vi "UpdateProject.vi"(8 "error in (no error)":errorcluster, 11 "DB_SQLite in":refnum<class "DB_SQLite.lvclass">) -> (0 "error out":errorcluster, 3 "DB_SQLite out":refnum<class "DB_SQLite.lvclass">)   [LabVIEW 2020, in "DB_SQLite.lvclass"]
uses:
  DB_SQLite.lvclass
  C:/dev/TRANCON/Classes/DB/DB.lvclass
  DB.lvclass/DB.ctl
  <vilib>/drjdpowell/SQLite Library/SQL Statement/SQL Statement.lvclass/SQL Statement.ctl
  <vilib>/drjdpowell/SQLite Library/SQL Statement/Bind Text.vi
  <vilib>/drjdpowell/SQLite Library/SQL Statement/Step.vi
  <vilib>/drjdpowell/SQLite Library/SQL Statement/Error Message.vi
  <vilib>/drjdpowell/SQLite Library/SQL Connection/Connection.lvclass
  <vilib>/drjdpowell/SQLite Library/SQL Statement/SQL Statement.lvclass
  <vilib>/drjdpowell/SQLite Library/Transaction Helpers/Transaction.lvlib
  DB.lvclass
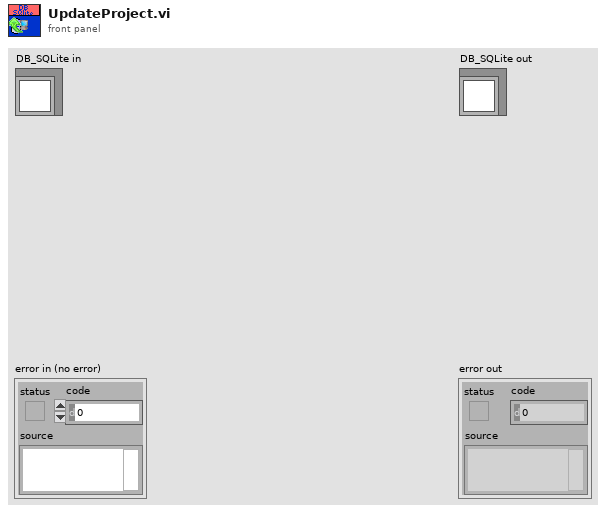
[diagram p1: front panel]
types:
  T1 = typedef "DB.lvclass/Def_DB_FP_ref_commands.ctl" = cluster{"Project Name":refnum<vi>, "Projects":refnum<vi>, "Project Description":refnum<vi>, "Project Date":refnum<vi>, "Project Users":refnum<vi>, "Samples":refnum<vi>, "Sample Name":refnum<vi>, "Sample Description":refnum<vi>, "Sample Date":refnum<vi>, "Experiments":refnum<vi>, "Exp Name":refnum<vi>, "Exp Description":refnum<vi>, "Exp Date":refnum<vi>, "Users":refnum<vi>, "User Name":refnum<vi>, "User Description":refnum<vi>, "User Date":refnum<vi>}
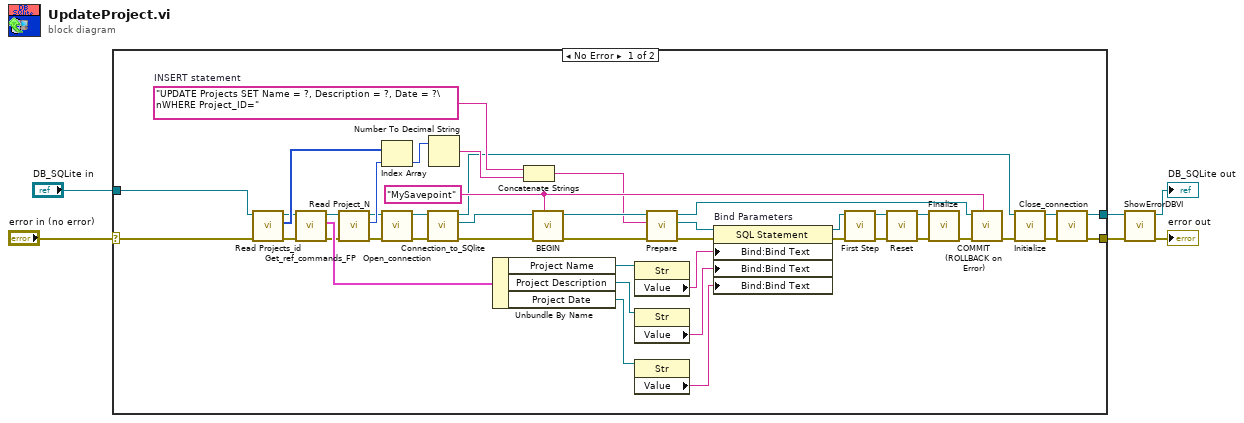
[diagram p0: block diagram]
diagram:
  n1 = case shown="No Error" "error in (no error)" {
    selector: "error in (no error)" -> [w19 w52]
    tunnel: [w12 w52] -> w3
    tunnel: [w11 w51] -> w4
    tunnel: "DB_SQLite in" -> [w23 w51]
    frame No Error {
      w44 = "MySavepoint" ("Savepoint name")
      w36 = "UPDATE Projects SET Name = ?, Description = ?, Date = ?\nWHERE Project_ID="  # INSERT statement
      n2 = call "Read Projects_id.vi"("error in (no error)"=w19, "DB in"=w23) -> ("error out"=w20:errorcluster, "Projects_id"=w22:i32[], "DB out"=w21:refnum<class "DB_SQLite.lvclass">)  [unwired: 7 in]
      n3 = call "Get_ref_commands_FP.vi"("error in (no error)"=w20, "DB in"=w21) -> ("error out"=w24:errorcluster, "controls_refs"=w25:T1, "DB out"=w26:refnum<class "DB_SQLite.lvclass">)  [unwired: 7 in]
      n4 = call "Read Project_N.vi"("error in (no error)"=w24, "DB in"=w26) -> ("error out"=w15:errorcluster, "Project_N"=w37:i16, "DB out"=w14:refnum<class "DB_SQLite.lvclass">)  [unwired: 7 in]
      n5 = Index Array(array=w22, index=w37) -> (element=w34:i32)
      n6 = call-dynamic "Open_connection.vi"("error in (no error)"=w15, "DB_SQLite in"=w14) -> ("error out"=w16:errorcluster, "DB_SQLite out"=w17:refnum<class "DB_SQLite.lvclass">)  [unwired: 8 in]
      n7 = call "Connection_to_SQlite.vi"("error in (no error)"=w16, "DB_SQLite in"=w17) -> ("error out"=w13:errorcluster, "SQlite connection"=w18:refnum<class "Connection.lvclass">, "DB_SQLite out"=w8:refnum<class "DB_SQLite.lvclass">)  [unwired: 7 in]
      n8 = Number To Decimal String(number=w34) -> (decimal integer string=w33:string)  [unwired: 1 in]
      n9 = Unbundle By Name(w25) -> ("Project Name"=w32:refnum<vi>, "Project Description"=w31:refnum<vi>, "Project Date"=w30:refnum<vi>)
      n10 = Concatenate Strings(w36, w33) -> (w35:string)
      n11 = call <vilib>:"BEGIN.vi"("Savepoint name"=w44, "error in (no error)"=w13, "SQLite Connection in"=w18) -> ("error out"=w45:errorcluster, "SQLite Connection"=w46:refnum<class "Connection.lvclass">)  [unwired: 7 in]
      n12 = property class="Str"(reference=w32) -> ("Value"=w29:string)  [unwired: 1 in, 2 out]
      n13 = property class="Str"(reference=w31) -> ("Value"=w28:string)  [unwired: 1 in, 2 out]
      n14 = property class="Str"(reference=w30) -> ("Value"=w27:string)  [unwired: 1 in, 2 out]
      n15 = call <vilib>:"Prepare.vi"("error in (no error)"=w45, "SQL"=w35, "SQLite Connection in"=w46) -> ("error out"=w49:errorcluster, "SQL Statement"=w50:refnum<class "SQL Statement.lvclass">, "SQLite Connection"=w43:refnum<class "Connection.lvclass">)  [unwired: 4 in, 2 out]
      n16 = property on="Bind Parameters" class="SQL Statement"(reference=w50, error in=w49, "Bind:Bind Text"=w29, "Bind:Bind Text"=w28, "Bind:Bind Text"=w27) -> (reference out=w41:refnum<class "SQL Statement.lvclass">, error out=w40:errorcluster)
      n17 = call <vilib>:"First Step.vi"("error in (no error)"=w40, "SQL Statement in"=w41) -> ("error out"=w39:errorcluster, "SQL Statement"=w38:refnum<class "SQL Statement.lvclass">)  [unwired: 7 in, 1 out]
      n18 = call <vilib>:"Reset.vi"("error in (no error)"=w39, "SQL Statement in"=w38) -> ("error out"=w47:errorcluster, "SQL Statement"=w48:refnum<class "SQL Statement.lvclass">)  [unwired: 8 in]
      n19 = call <vilib>:"Finalize.vi"("error in (no error)"=w47, "SQL Statement in"=w48) -> ("error out"=w42:errorcluster)  [unwired: 9 in]
      n20 = call <vilib>:"COMMIT (ROLLBACK on Error).vi"("Savepoint name"=w44, "error in (no error)"=w42, "SQLite Connection in"=w43) -> ("error out"=w9:errorcluster)  [unwired: 7 in, 1 out]
      n21 = call "Initialize.vi"("error in (no error)"=w9, "DB in"=w8) -> ("error out"=w10:errorcluster, "DB out"=w7:refnum<class "DB_SQLite.lvclass">)  [unwired: 8 in]
      n22 = call-dynamic "Close_connection.vi"("error in (no error)"=w10, "DB_SQLite in"=w7) -> ("error out"=w12:errorcluster, "DB_SQLite out"=w11:refnum<class "DB_SQLite.lvclass">)  [unwired: 8 in]
    }
    frame Error {
    }
  }
  n23 = call "ShowErrorDBVI.vi"("error in (no error)"=w3, "DB in"=w4) -> ("error out"=→"error out":errorcluster, "DB out"=→"DB_SQLite out":refnum<class "DB_SQLite.lvclass">)  [unwired: 8 in]
